vi "TurnToDegrees.vi"(9 "Speed":dbl=0.6, 10 "RobotDriveDevRef":T1, 11 "Angle":dbl) -> ()   [LabVIEW 2017]
uses:
  <vilib>/Rock Robotics/WPI/RobotDrive/WPI_RobotDriveDevRef.ctl
  <vilib>/Rock Robotics/WPI/MotorControl/WPI_MotorControlDeviceRef.ctl
  <vilib>/Rock Robotics/WPI/MotorControl/WPI_MotorControlType.ctl
  <vilib>/Rock Robotics/SystemInterfaces/DIO/FPGA_DIOPWMChannel.ctl
  <vilib>/Rock Robotics/WPI/PWM/WPI_PWMDeadband.ctl
  <vilib>/Rock Robotics/SystemInterfaces/DIO/FPGA_DIOChannel.ctl
  Robot Global Data.vi
  <vilib>/Rock Robotics/WPI/RobotDrive/WPI_RobotDriveArcadeDrive_Standard(NoSaturation).vi
  <vilib>/addons/control/pid/pid.llb/PID (DBL).vi
  <vilib>/addons/control/pid/NI_PID_pid.lvlib
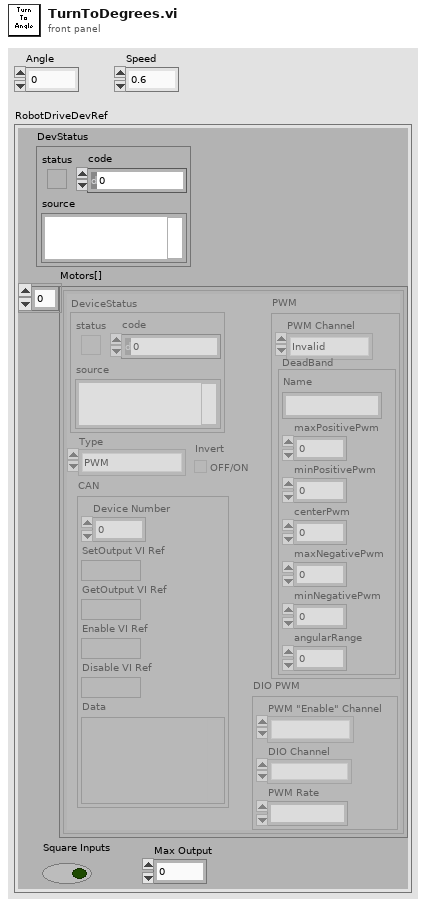
[diagram p1: front panel]
types:
  T1 = typedef "WPI_RobotDriveDevRef.ctl" = cluster{"DevStatus":errorcluster, "Motors[]":T2[], "Square Inputs":bool, "Max Output":dbl}
  T2 = typedef "WPI_MotorControlDeviceRef.ctl" = cluster{"DeviceStatus":errorcluster, "Type":T3, "PWM":cluster{"PWM Channel":T4, "DeadBand":T5}, "CAN":cluster{"Device Number":u8, "SetOutput VI Ref":variant, "GetOutput VI Ref":variant, "Enable VI Ref":variant, "Disable VI Ref":variant, "Data":variant}, "Invert":bool, "DIO PWM":cluster{"PWM \"Enable\" Channel":T4, "DIOChannel":T6, "PWM Rate":dbl}}
  T3 = typedef "WPI_MotorControlType.ctl" = enum16{"PWM", "CAN", "DIO PWM"}
  T4 = typedef "FPGA_DIOPWMChannel.ctl" = enum8{"PWM 0", "PWM 1", "PWM 2", "PWM 3", "PWM 4", "PWM 5", "PWM 6", "PWM 7", "PWM 8", "PWM 9", "PWM MXP 0", "PWM MXP 1", "PWM MXP 2", "PWM MXP 3", "PWM MXP 4", "PWM MXP 5", "PWM MXP 6", "PWM MXP 7", "PWM MXP 8", "PWM MXP 9", "Invalid"}
  T5 = typedef "WPI_PWMDeadband.ctl" = cluster{"Name":string, "maxPositivePwm":i32, "minPositivePwm":i32, "centerPwm":i32, "maxNegativePwm":i32, "minNegativePwm":i32, "angularRange":u16}
  T6 = typedef "FPGA_DIOChannel.ctl" = enum8{"DIO 0", "DIO 1", "DIO 2", "DIO 3", "DIO 4", "DIO 5", "DIO 6", "DIO 7", "DIO 8", "DIO 9", "DIO MXP 0", "DIO MXP 1", "DIO MXP 2", "DIO MXP 3", "DIO MXP 4", "DIO MXP 5", "DIO MXP 6", "DIO MXP 7", "DIO MXP 8", "DIO MXP 9", "DIO MXP 10", "DIO MXP 11", "DIO MXP 12", "DIO MXP 13", "DIO MXP 14", "DIO MXP 15", "SPI Port CS1", "SPI Port CS2", "SPI Port CS3", "SPI Port MISO", "SPI Port MOSI", "Invalid"}
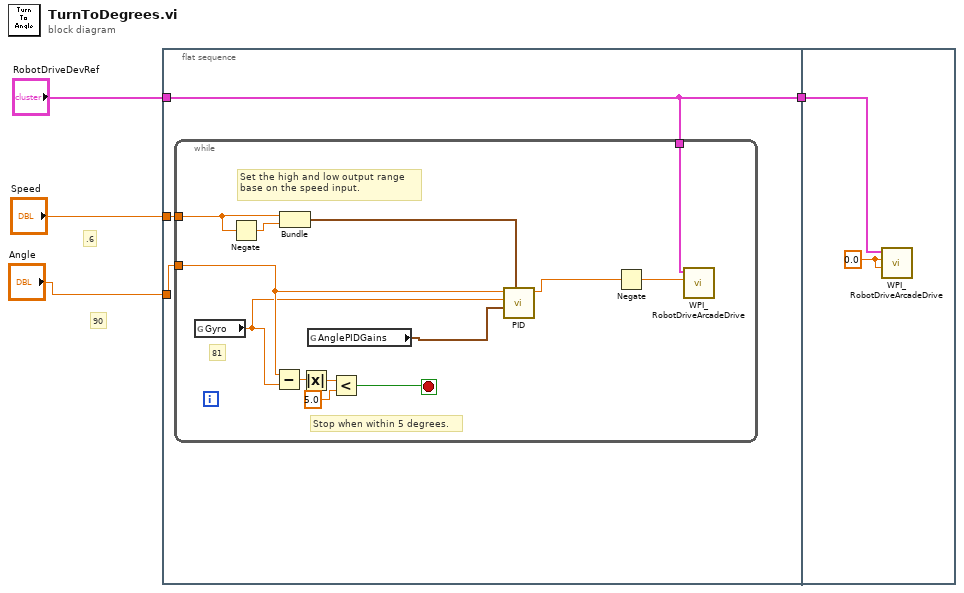
[diagram p0: block diagram]
diagram:
  # "90"
  # ".6"
  n1 = flat-sequence {
    tunnel: "Speed" -> [w7]
    tunnel: "Angle" -> [w6]
    tunnel: [w5] -> w2
    tunnel: "RobotDriveDevRef" -> [w5]
    tunnel: w2 -> [w21]
    frame #0 {
      n2 = while {
        tunnel: w6 -> [w13]
        tunnel: w7 -> [w16]
        tunnel: w5 -> [w8]
        stop <- w11 stop-if-true
        # "Stop when within 5 degrees."
        # "Set the high and low output range\nbase on the speed input."
        # "81"
        n3 = global read "Robot Global Data.vi" "Gyro"() -> (w12:dbl)
        n4 = Negate(x=w16) -> (-x=w17:dbl)
        n5 = Subtract(x=w13, y=w12) -> (x-y=w20:dbl)
        n6 = Bundle("Speed"=w16, w17) -> (w15:cluster{"Speed":dbl, dbl})  [unwired: 1 in]
        n7 = Absolute Value(x=w20) -> (abs(x)=w19:dbl)
        n8 = global read "Robot Global Data.vi" "AnglePIDGains"() -> (w14:cluster{"P":dbl, "I":dbl, "D":dbl})
        n9 = Less?(x=w19, y=5.0) -> (x < y?=w11:bool)
        n10 = call-poly <vilib>:"PID.vi"("output range"=w15, "PID gains"=w14, "process variable"=w12, "setpoint"=w13) -> ("output"=w10:dbl)  [unwired: 6 in, 1 out]
        n11 = Negate(x=w10) -> (-x=w9:dbl)
        n12 = call-poly <vilib>:"WPI_RobotDriveArcadeDrive.vi"("X axis value"=w9, "RobotDriveDevRef"=w8) -> ()  [unwired: 7 in, 3 out]
      }
    }
    frame #1 {
      w22 = 0.0 ("X axis value")
      n13 = call-poly <vilib>:"WPI_RobotDriveArcadeDrive.vi"("Y axis value"=w22, "X axis value"=w22, "RobotDriveDevRef"=w21) -> ()  [unwired: 6 in, 3 out]
    }
  }
